vi "LightField_configuration_test.vi"() -> ()   [LabVIEW 2020]
uses:
  LightField Automation.lvclass
panel:
  in  "Boolean":bool
  out "ROI 1, Frame 1, Row 1":dbl[](graph)
  out "ROI 1, Frame 1":dbl[][](graph)
  out "Data":T1(array[cluster])
  in  "stop":bool
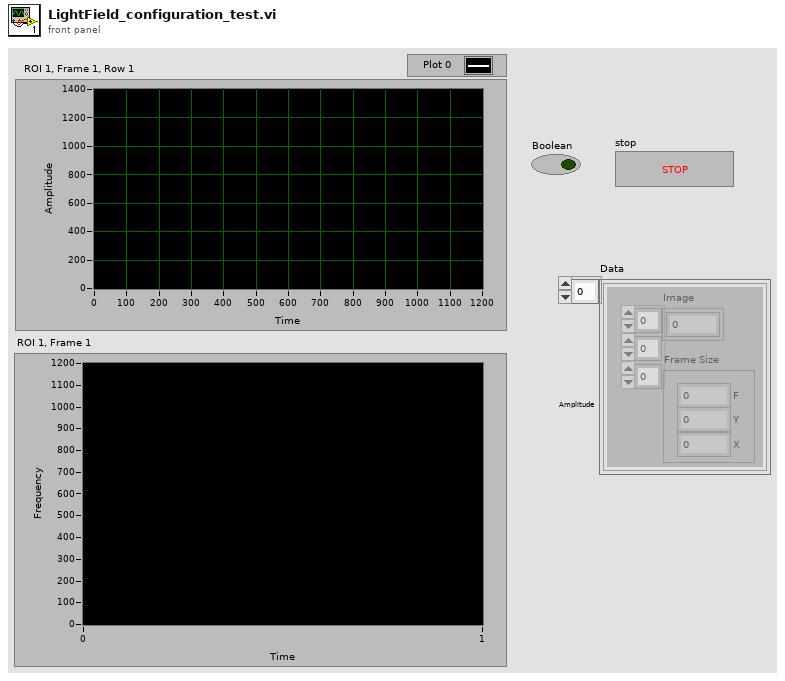
[diagram p1: front panel]
types:
  T1 = cluster{"Image":dbl[][][], "Frame Size":cluster{"F":i32, "Y":i32, "X":i32}}[]
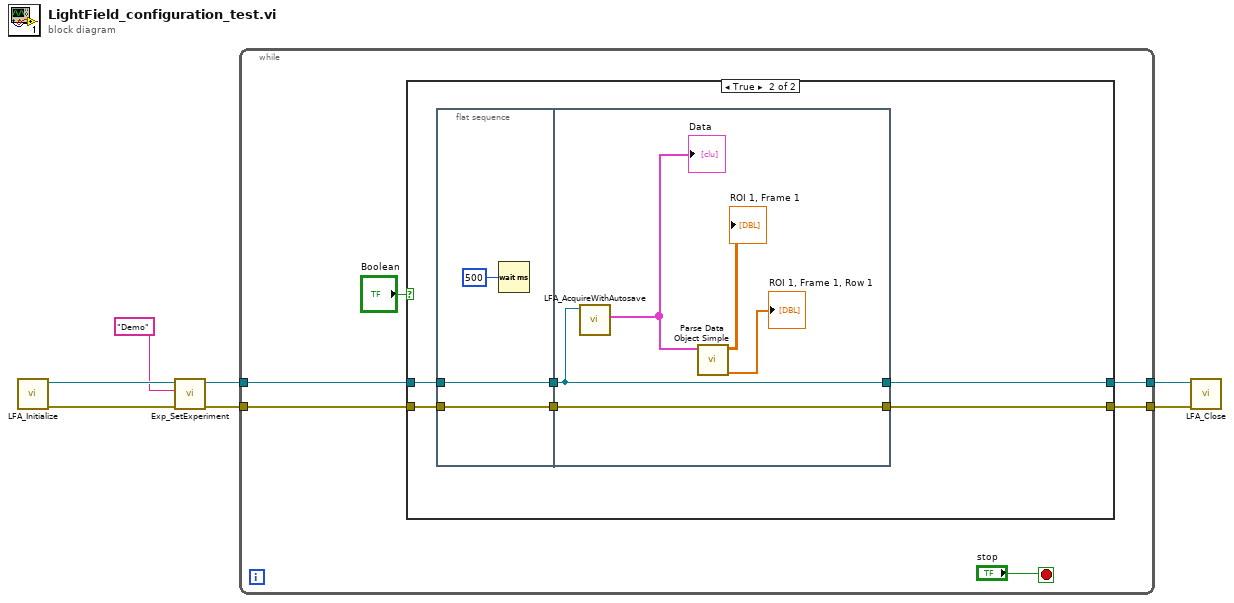
[diagram p0: block diagram]
diagram:
  n1 = call "LFA_Initialize.vi"() -> ("error out"=w7:errorcluster, "LightField Automation out"=w6:refnum<class "LightField Automation.lvclass">)  [unwired: 10 in]
  n2 = call "Exp_SetExperiment.vi"("error in (no error)"=w7, "ExperimentName"="Demo", "LightField Automation in"=w6) -> ("error out"=w4:errorcluster, "LightField Automation out"=w3:refnum<class "LightField Automation.lvclass">)  [unwired: 7 in]
  n3 = while {
    tunnel: w4 -> [w13]
    tunnel: w3 -> [w12]
    tunnel: [w10] -> w2
    tunnel: [w9] -> w1
    stop <- "stop" stop-if-true
    n4 = case shown="True" "Boolean" {
      tunnel: w13 -> [w14 w16]
      tunnel: w12 -> [w15 w17]
      tunnel: [w14 w19] -> w10
      tunnel: [w15 w18] -> w9
      frame False {
      }
      frame True {
        n5 = flat-sequence {
          tunnel: [w22] -> w21
          tunnel: [w23] -> w20
          tunnel: w17 -> [w23]
          tunnel: w16 -> [w22]
          tunnel: [w25] -> w18
          tunnel: [w29] -> w19
          tunnel: w21 -> [w29]
          tunnel: w20 -> [w25]
          frame #0 {
            n6 = Wait (ms)(milliseconds to wait=u32 500 ("millisecond timer value")) -> ()  [unwired: 1 out]
          }
          frame #1 {
            n7 = call "LFA_AcquireWithAutosave.vi"("LightField Automation in"=w25) -> ("Data"=w28:T1)  [unwired: 8 in, 2 out]
            "Data" <- w28
            n8 = call "Parse Data Object Simple.vi"("Data"=w28) -> ("ROI 1, Frame 1, Row 1"=→"ROI 1, Frame 1, Row 1":dbl[], "ROI 1, Frame 1"=→"ROI 1, Frame 1":dbl[][])  [unwired: 9 in]
          }
        }
      }
    }
  }
  n9 = call "LFA_Close.vi"("error in (no error)"=w2, "LightField Automation in"=w1) -> ()  [unwired: 8 in, 2 out]
